vi "SD-Component Generator.vi"(1 "Component definition":T1={"First color"=0, "Last color"=0, "Middle color"=0, "Middle #"=2}) -> (0 "Component array":u8[](array[numeric]))   [LabVIEW 2020]
doc: "Component Generator.vi is a subVI called by Color Table Generator.vi.\n\nThis VI calculates a range of colors based on initial, middle and final colors. The middle color can be specified at any location within the array. It doesn't have to be the middle index of the array."
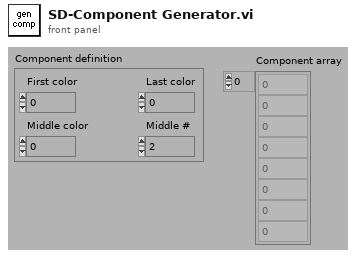
[diagram p1: front panel]
types:
  T1 = cluster{"First color":u8, "Last color":u8, "Middle color":u8, "Middle #":u8}
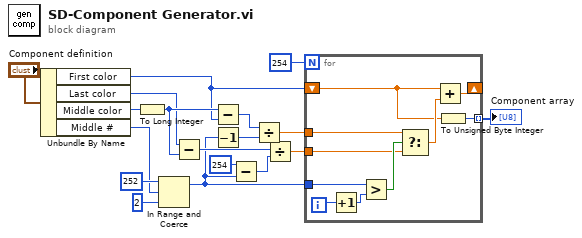
[diagram p0: block diagram]
diagram:
  n1 = Unbundle By Name("Component definition") -> ("First color"=w7:u8, "Last color"=w6:u8, "Middle color"=w5:u8, "Middle #"=w2:u8)
  n2 = To Long Integer(number=w5) -> (32bit integer=w11:i32)
  n3 = In Range and Coerce(upper limit=u8 252, x=w2, lower limit=u8 2) -> (coerced(x)=w1:u8)  [unwired: 1 out]
  n4 = Subtract(x=w6, y=w11) -> (x-y=w9:i32)
  n5 = Subtract(x=w11, y=w7) -> (x-y=w10:i32)
  n6 = Decrement(x=w1) -> (x-1=w17:u8)
  n7 = Subtract(x=u8 254, y=w1) -> (x-y=w15:u8)
  n8 = Divide(x=w10, y=w17) -> (x/y=w14:dbl)
  n9 = Divide(x=w9, y=w15) -> (x/y=w13:dbl)
  n10 = for {
    N: 254 -> [_]
    tunnel: w1 -> [w28]
    shift-right: [w21] -> _
    shift-left: w7 -> [w23]
    tunnel: w14 -> [w25]
    tunnel: w13 -> [w24]
    tunnel: [w22] -> w12 mode=indexing
    i -> [w20]
    n11 = Increment(x=w20) -> (x+1=w19:i32)
    n12 = Greater?(x=w28, y=w19) -> (0:w27:bool)
    n13 = Select(t=w25, s=w27, f=w24) -> (s? t:f=w26:dbl)
    n14 = Add(x=w23, y=w26) -> (x+y=w21:dbl)
    n15 = To Unsigned Byte Integer(number=w23) -> (unsigned 8bit integer=w22:u8)
  }
  "Component array" <- w12
